vi "FRCts20_Backend_Event_GET_return.vi"(7 "Event":T1, 8 "error in (no error)":errorcluster, 11 "recordset data":variant[][](array[variant])) -> (0 "error out":errorcluster, 3 "data string":string)   [LabVIEW 2014, in "FRCts20_Backend_Engine.lvlib"]
doc: "Parses and returns the specific team's data"
uses:
  FRCts20_Backend_Engine.lvlib
  FRCts20_Backend_API/Event.ctl
  FRCts20_Backend_API/ApiReturn.ctl
  FRCts20_Backend_API/EventRoot.ctl
  FRCts20_Backend_API/TeamRoot.ctl
  FRCts20_Backend_API/FRCts20_Backend_API_SW.ctl
  <vilib>/addons/database/_DB Variant To Data/Database Variant To Data.xnode
  FRCts20_Backend_API/FRCts20_Backend_API.lvlib
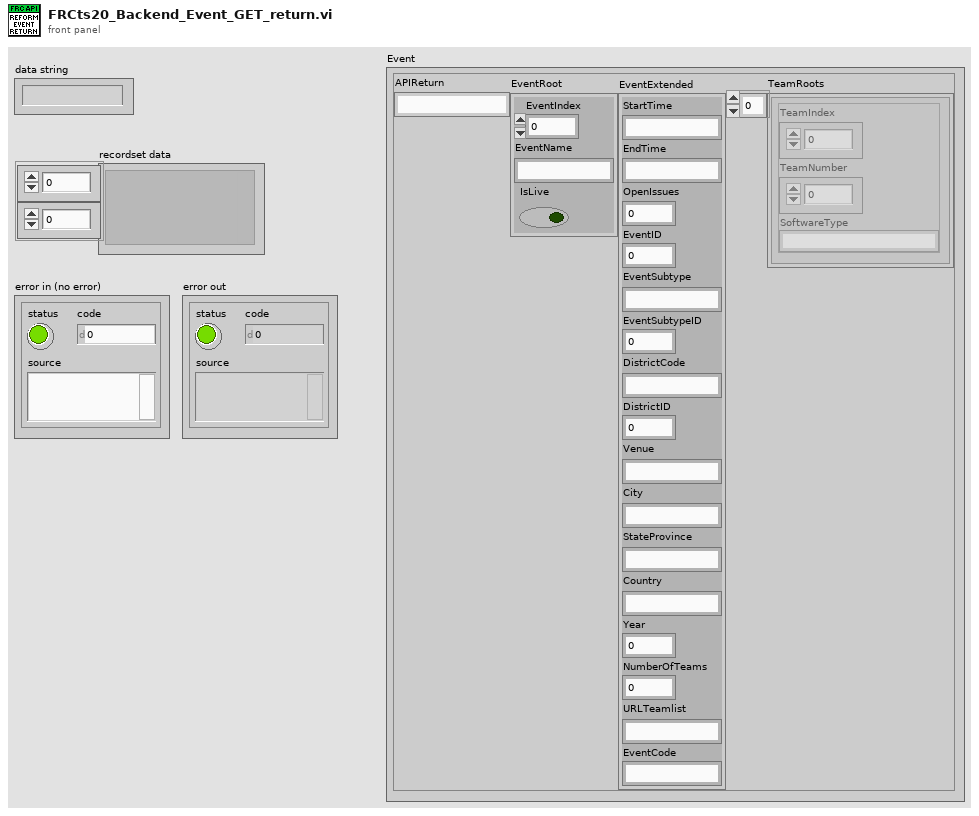
[diagram p1: front panel]
types:
  T1 = typedef "FRCts20_Backend_Engine.lvlib/FRCts20_Backend_API.lvlib/Event.ctl" = cluster{"APIReturn":T2, "EventRoot":T3, "EventExtended":cluster{"StartTime":string, "EndTime":string, "OpenIssues":u8, "EventID":u32, "EventSubtype":string, "EventSubtypeID":u32, "DistrictCode":string, "DistrictID":u32, "Venue":string, "City":string, "StateProvince":string, "Country":string, "Year":u32, "NumberOfTeams":u32, "URLTeamlist":string, "EventCode":string}, "TeamRoots":T4[]}
  T2 = typedef "FRCts20_Backend_Engine.lvlib/FRCts20_Backend_API.lvlib/ApiReturn.ctl" = string
  T3 = typedef "FRCts20_Backend_Engine.lvlib/FRCts20_Backend_API.lvlib/EventRoot.ctl" = cluster{"EventIndex":i32, "EventName":string, "IsLive":bool}
  T4 = typedef "FRCts20_Backend_Engine.lvlib/FRCts20_Backend_API.lvlib/TeamRoot.ctl" = cluster{"TeamIndex":i32, "TeamNumber":u32, "SoftwareType":T5}
  T5 = typedef "FRCts20_Backend_Engine.lvlib/FRCts20_Backend_API.lvlib/FRCts20_Backend_API_SW.ctl" = string
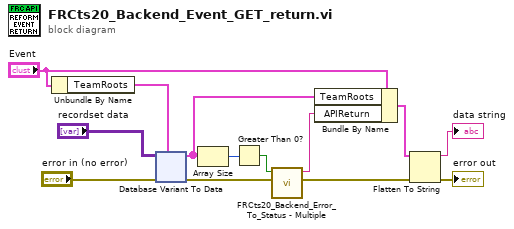
[diagram p0: block diagram]
diagram:
  n1 = Unbundle By Name("Event") -> ("TeamRoots"=w3:T4[])
  n2 = xnode "Database Variant To Data"("database variant"="recordset data", "error in (no error)"="error in (no error)", "type"=w3) -> ("data"=w1:T4[], "error out"=w8:errorcluster)
  n3 = Array Size(array=w1) -> (size(s)=w6:i32)
  n4 = Greater Than 0?(x=w6) -> (x > 0?=w4:bool)
  n5 = call "FRCts20_Backend_Error_To_Status - Multiple.vi"("error in (no error)"=w8, "rows affected?"=w4) -> ("error out"=w7:errorcluster, "String"=w12:string)  [unwired: 8 in]
  n6 = Bundle By Name(cluster="Event", "TeamRoots"=w1, "APIReturn"=w12) -> (w10:T1)
  n7 = Flatten To String(anything=w10, error in (no error)=w7) -> (data string=→"data string":string, error out=→"error out":errorcluster)  [unwired: 2 in, 1 out]
